vi "WaveformWriter.vi"() -> ()   [LabVIEW 2020]
doc: "Copyright © 2008 - 2024 VI Technologies B.V. \nALL RIGHTS RESERVED"
uses:
  SuperNS/StreamStatus.ctl
  SuperNS/SuperNS.lvclass
  WaveFormData/WfmData.lvclass
panel:
  out "error out":errorcluster
  out "StreamStatus":T1
  out "My IP address":string
  in  "EnableWaveformGen":bool
  in  "My Name":string="DataWriter"
  in  "Reader URL":string="//localhost/DataReader"
  # "Waveform writer"
  # "Copyright (c) 2024, VI Technologies B.V.\nAll rights reserved.\n\nRedistribution and use in source and binary forms, with or without modification, are permitted provided that \nthe following conditions are met:\n\n * Redistributions of source code must retain the above copyright notice, this list of conditions and the \nfollowing disclaimer.\n * Redistributions in binary form must reproduce the above copyright notice, this list of conditions and the \nfollowing disclaimer in the documentation and/or other materials provided with the distribution.\n * Neither the name of VI Technologies B.V. nor the names of its contributors may be used to endorse or \npromote products derived from this software without specific prior written permission.\n\nTHIS SOFTWARE IS PROVIDED BY THE COPYRIGHT HOLDERS AND CONTRIBUTORS \"AS IS\" AND ANY EXPRESS OR \nIMPLIED WARRANTIES, INCLUDING, BUT NOT LIMITED TO, THE IMPLIED WARRANTIES OF MERCHANTABILITY \nAND FITNESS FOR A PARTICULAR PURPOSE ARE DISCLAIMED. IN NO EVENT SHALL THE COPYRIGHT OWNER OR \nCONTRIBUTORS BE LIABLE FOR ANY DIRECT, INDIRECT, INCIDENTAL, SPECIAL, EXEMPLARY, OR CONSEQUENTIAL \nDAMAGES (INCLUDING, BUT NOT LIMITED TO, PROCUREMENT OF SUBSTITUTE GOODS OR SERVICES; LOSS OF \nUSE, DATA, OR PROFITS; OR BUSINESS INTERRUPTION) HOWEVER CAUSED AND ON ANY THEORY OF LIABILITY, \nWHETHER IN CONTRACT, STRICT LIABILITY, OR TORT (INCLUDING NEGLIGENCE OR OTHERWISE) ARISING IN ANY \nWAY OUT OF THE USE OF THIS SOFTWARE, EVEN IF ADVISED OF THE POSSIBILITY OF SUCH DAMAGE.\n\nFor more information, please visit https://www.vi-tech.nl or contact us at info@vi-tech.nl"
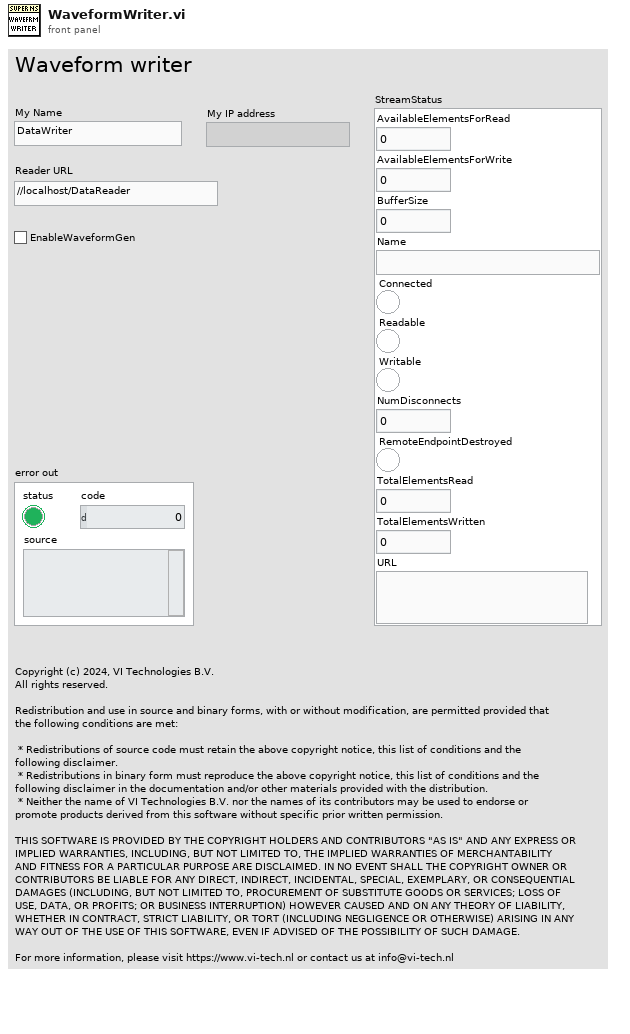
[diagram p1: front panel]
types:
  T1 = typedef "SuperNS.lvclass/StreamStatus.ctl" = cluster{"AvailableElementsForRead":i32, "AvailableElementsForWrite":i32, "BufferSize":i32, "Name":string, "Connected":bool, "Readable":bool, "Writable":bool, "NumDisconnects":u32, "RemoteEndpointDestroyed":bool, "TotalElementsRead":u64, "TotalElementsWritten":u64, "URL":string}
  T2 = enum16{"None (High througput mode)", "All Elements Read From Stream", "All Elements Available for Reading"}
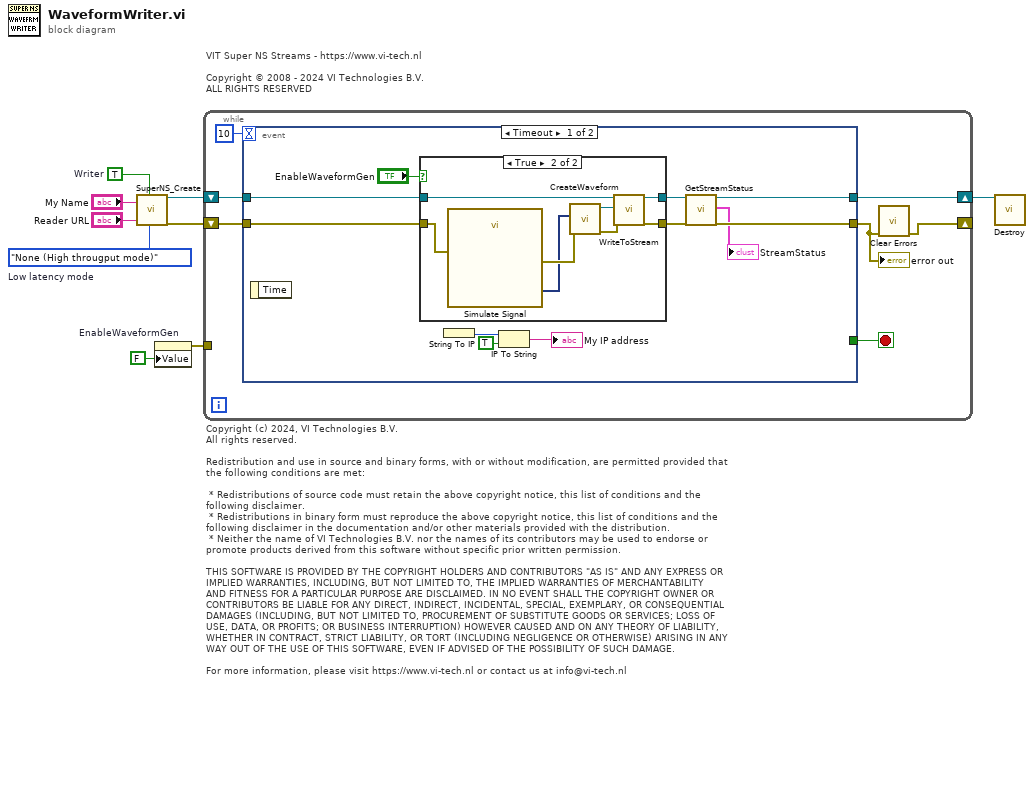
[diagram p0: block diagram]
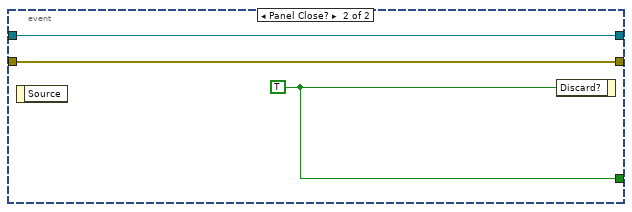
[diagram p3: hidden frame]
diagram:
  w4 = T2."None (High througput mode)"  # Low latency mode
  w1 = TRUE  # Writer
  # "VIT Super NS Streams - https://www.vi-tech.nl\n\nCopyright © 2008 - 2024 VI Technologies B.V. \nALL RIGHTS RESERVED"
  # "Copyright (c) 2024, VI Technologies B.V.\nAll rights reserved.\n\nRedistribution and use in source and binary forms, with or without modification, are permitted provided that \nthe following conditions are met:\n\n * Redistributions of source code must retain the above copyright notice, this list of conditions and the \nfollowing disclaimer.\n * Redistributions in binary form must reproduce the above copyright notice, this list of conditions and the \nfollowing disclaimer in the documentation and/or other materials provided with the distribution.\n * Neither the name of VI Technologies B.V. nor the names of its contributors may be used to endorse or \npromote products derived from this software without specific prior written permission.\n\nTHIS SOFTWARE IS PROVIDED BY THE COPYRIGHT HOLDERS AND CONTRIBUTORS \"AS IS\" AND ANY EXPRESS OR \nIMPLIED WARRANTIES, INCLUDING, BUT NOT LIMITED TO, THE IMPLIED WARRANTIES OF MERCHANTABILITY \nAND FITNESS FOR A PARTICULAR PURPOSE ARE DISCLAIMED. IN NO EVENT SHALL THE COPYRIGHT OWNER OR \nCONTRIBUTORS BE LIABLE FOR ANY DIRECT, INDIRECT, INCIDENTAL, SPECIAL, EXEMPLARY, OR CONSEQUENTIAL \nDAMAGES (INCLUDING, BUT NOT LIMITED TO, PROCUREMENT OF SUBSTITUTE GOODS OR SERVICES; LOSS OF \nUSE, DATA, OR PROFITS; OR BUSINESS INTERRUPTION) HOWEVER CAUSED AND ON ANY THEORY OF LIABILITY, \nWHETHER IN CONTRACT, STRICT LIABILITY, OR TORT (INCLUDING NEGLIGENCE OR OTHERWISE) ARISING IN ANY \nWAY OUT OF THE USE OF THIS SOFTWARE, EVEN IF ADVISED OF THE POSSIBILITY OF SUCH DAMAGE.\n\nFor more information, please visit https://www.vi-tech.nl or contact us at info@vi-tech.nl"
  n1 = call "SuperNS_Create.vi"("NSName"="My Name", "RemoteEP_URL"="Reader URL", "Writer (F: Reader)"=w1, "Low latency mode"=w4) -> ("SuperNS Reference"=w2:refnum<class "SuperNS.lvclass">, "error out"=w8:errorcluster)  [unwired: 14 in]
  n2 = property on="EnableWaveformGen" class="Bool (strict)"("Value"=FALSE ("EnableWaveformGen")) -> (error out=w9:errorcluster)  [unwired: 2 in, 1 out]
  n3 = while {
    shift-right: [w12] -> w6
    shift-left: w2 -> [w13]
    shift-right: [w15] -> _
    shift-left: w8 -> [w16]
    tunnel: w9 -> [_]
    stop <- w14 stop-if-true
    n4 = event shown="[0] Timeout" {
      selector: _ -> [_ _]
      dyn-events: _ -> [_ _]
      timeout: 10 -> [_ _]
      tunnel: [_ w40] -> w14
      tunnel: [w22 w39] -> w12
      tunnel: w13 -> [w24 w39]
      tunnel: w16 -> [w18 w38]
      tunnel: [w26 w38] -> w10
      event Timeout {
        n5 = event-data() -> ()  [unwired: 1 in, 1 out]
        n6 = case shown="True" "EnableWaveformGen" {
          tunnel: w24 -> [w29 w35]
          tunnel: [w29 w36] -> w23
          tunnel: [w28 w37] -> w27
          tunnel: w18 -> [w28 w30]
          frame False {
          }
          frame True {
            n7 = call "Simulate Signal"("error in (no error)"=w30) -> ("Sine"=w31:dynamicdata, "error out"=w33:errorcluster)  [unwired: 13 in]
            n8 = call "CreateWaveform.vi"("error in"=w33, "Waveform"=w31) -> ("error out"=w32:errorcluster, "MsgData out"=w34:refnum<class "WfmData.lvclass">)  [unwired: 8 in]
            n9 = call-dynamic "WriteToStream.vi"("reference in"=w35, "LabVIEW Object"=w34, "error in"=w32) -> ("reference out"=w36:refnum<class "SuperNS.lvclass">, "error out"=w37:errorcluster)  [unwired: 14 in, 1 out]
          }
        }
        n10 = String To IP() -> (0:w21:u32)  [unwired: 1 in]
        n11 = IP To String(1:TRUE ("dot notation? (F)"), 2:w21) -> (0:→"My IP address":string)
        n12 = call-dynamic "GetStreamStatus.vi"("reference in"=w23, "error in"=w27) -> ("reference out"=w22:refnum<class "SuperNS.lvclass">, "StreamStatus"=→"StreamStatus":T1, "error out"=w26:errorcluster)  [unwired: 13 in, 2 out]
      }
      event Panel Close? {
        w40 = TRUE ("Discard?")
        n13 = event-data() -> ()  [unwired: 1 in, 1 out]
        n14 = event-data("Discard?"=w40) -> ()  [unwired: 1 in, 1 out]
      }
    }
    "error out" <- w10
    n15 = call <vilib>:"Clear Errors.vi"("error in (no error)"=w10) -> ("error out"=w15:errorcluster)  [unwired: 5 in, 1 out]
  }
  n16 = call-dynamic "Destroy.vi"("reference in"=w6) -> ()  [unwired: 17 in, 2 out]
